vi "WPI_GyroAnalogOpen.vi"(6 "Calibrated Center Voltage":dbl, 7 "Calibration Time (s)":dbl=2.0, 8 "error in (no error)":errorcluster, 9 "Calibrate On Open":bool=TRUE, 10 "Analog Channel":T1) -> (0 "error out":errorcluster, 2 "Calibrated Center Voltage Out":dbl, 3 "GyroDevRef":T2={"DevStatus"={"status"=FALSE, "code"=0, "source"=""}, "Analog Channel"=enum."AI 1", "Gain (VoltsPerDegree/Second)"=0.0, "Gyro Type"=enum."Analog", "Handle"=0, "SPI Bus"=enum."Invalid", "Device Found"=FALSE, "Sample Rate"=1.0, "Calibrate On Open"=FALSE, "Offset"=0.0} {"Sample Rate" min=0.25 max=100.0 step=0.25})   [LabVIEW 2017]
doc: "Opens a reference to the gyroscope you specify. You must open a reference before using any other VIs on this palette.\n\nThis software is licensed. Open the labview\\readme\\WPI Robotics Library Open Source License.txt file for more information."
uses:
  <vilib>/Rock Robotics/WPI/Gyro/WPI_GyroDevRef.ctl
  <vilib>/Rock Robotics/SystemInterfaces/AI/FPGA_AIChannel.ctl
  <vilib>/Rock Robotics/SystemInterfaces/spilib/spi_bus.ctl
  <vilib>/Rock Robotics/SystemInterfaces/AI/FPGA_AIGyroChannel.ctl
  <vilib>/robotics/Simulator/Engine/ctl/DeviceID.ctl
  <instrlib>/Sparkfun Atomic IMU/HAIOL/Simulator/Sparkfun Atomic IMU Simulator.lvclass
  <vilib>/robotics/Simulator/NI_Robotics_Simulator.lvlib
  <instrlib>/Honeywell Compass HMC6343/HAIOL/Simulator/Honeywell Compass HMC6343 Simulator.lvclass
panel:
  # "Analog"
  # "XRS"
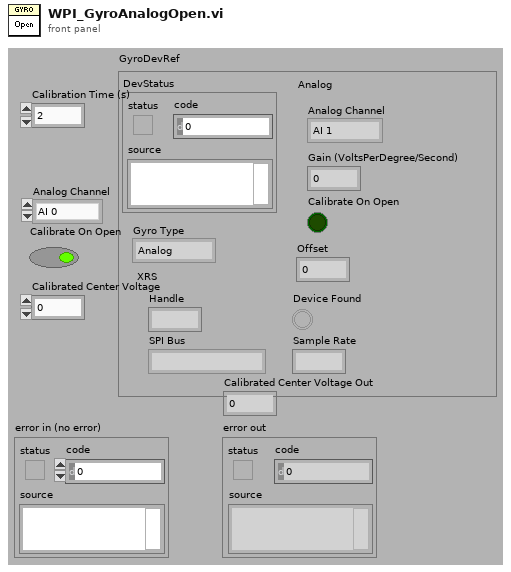
[diagram p1: front panel]
types:
  T1 = typedef "FPGA_AIGyroChannel.ctl" = enum8{"AI 0", "AI 1", "Invalid"}
  T2 = typedef "WPI_GyroDevRef.ctl" = cluster{"DevStatus":errorcluster, "Analog Channel":T3, "Gain (VoltsPerDegree/Second)":dbl, "Gyro Type":enum16{"Analog", "XRS450"}, "Handle":i32, "SPI Bus":T4, "Device Found":bool, "Sample Rate":dbl, "Calibrate On Open":bool, "Offset":dbl}
  T3 = typedef "FPGA_AIChannel.ctl" = enum8{"AI 0", "AI 1", "AI 2", "AI 3", "AI MXP 0", "AI MXP 1", "AI MXP 2", "AI MXP 3", "Invalid"}
  T4 = typedef "spi_bus.ctl" = enum16{"SPI On-Board, CS0", "SPI On-Board, CS1", "SPI On-Board, CS2", "SPI On-Board, CS3", "SPI MXP", "Invalid"}
  T5 = typedef "NI_Robotics_Simulator.lvlib/DeviceID.ctl" = cluster{"robot ID":string, "sensor/actuator ID":string}
  T6 = typedef "WPI_AnalogChannelDevRef.ctl" = cluster{"DevStatus":errorcluster, "Analog Channel":T3}
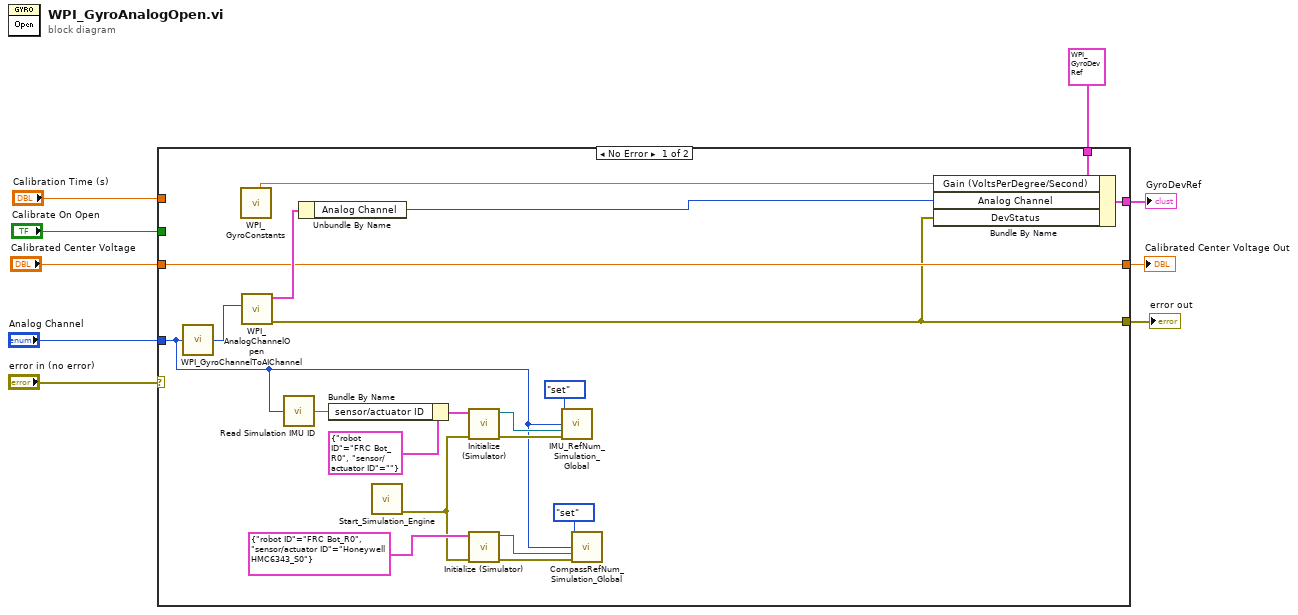
[diagram p0: block diagram]
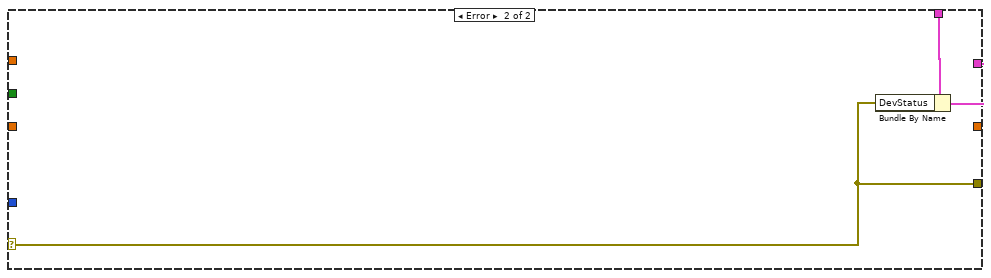
[diagram p2: hidden frame]
diagram:
  n1 = case shown="No Error" "error in (no error)" {
    selector: "error in (no error)" -> [_ w30]
    tunnel: "Analog Channel" -> [w15 _]
    tunnel: [w22 w30] -> w8
    tunnel: T2 {"DevStatus"={"status"=FALSE, "code"=0, "source"=""}, "Analog Channel"=enum."Invalid", "Gain (VoltsPerDegree/Second)"=0.0, "Gyro Type"=enum."Analog", "Handle"=0, "SPI Bus"=enum."Invalid", "Device Found"=FALSE, "Sample Rate"=1.0, "Calibrate On Open"=FALSE, "Offset"=0.0} ("GryoDevStatus") -> [w28 w31]
    tunnel: [w27 w32] -> w5
    tunnel: "Calibrate On Open" -> [_ _]
    tunnel: "Calibrated Center Voltage" -> [w23 _]
    tunnel: "Calibration Time (s)" -> [_ _]
    tunnel: [w23 _] -> w1
    frame No Error {
      n2 = call <vilib>:"WPI_GyroChannelToAIChannel.vi"("Gyro Channel"=w15) -> ("AI Channel"=w26:T3)  [unwired: 4 out]
      n3 = call <vilib>:"WPI_GyroConstants.vi"() -> ("Gain (VoltsPerDegreePerSecond)"=w24:dbl)  [unwired: 11 out]
      n4 = call <vilib>:"WPI_AnalogChannelOpen.vi"("Analog Channel"=w26) -> ("error out"=w22:errorcluster, "AIDeviceRef"=w25:T6)  [unwired: 2 in, 7 out]
      n5 = call <vilib>:"Read Simulation IMU ID.vi"("Analog Channel"=w15) -> ("gyro ID"=w19:string)  [unwired: 13 in, 1 out]
      n6 = Unbundle By Name(w25) -> ("Analog Channel"=w29:T3)
      n7 = Bundle By Name(cluster=T5 {"robot ID"="FRC Bot_R0", "sensor/actuator ID"=""} ("Device ID"), "sensor/actuator ID"=w19) -> (w20:T5)
      n8 = call <vilib>:"Start_Simulation_Engine.vi"() -> ("error out"=w13:errorcluster)  [unwired: 15 in]
      n9 = call <instrlib>:"Initialize (Simulator).vi"("error in (no error)"=w13, "Device ID"=w20) -> ("error out"=w16:errorcluster, "Sparkfun Atomic IMU out"=w18:refnum<class "Sparkfun Atomic IMU.lvclass">)  [unwired: 8 in]
      n10 = call <instrlib>:"Initialize (Simulator).vi"("error in (no error)"=w13, "Device ID"=T5 {"robot ID"="FRC Bot_R0", "sensor/actuator ID"="Honeywell HMC6343_S0"}) -> ("error out"=w11:errorcluster, "Honeywell Compass HMC6343"=w10:refnum<class "Honeywell Compass HMC6343.lvclass">)  [unwired: 8 in]
      n11 = call <vilib>:"IMU_RefNum_Simulation_Global.vi"("menu"=enum16{"set", "get", "delete"}."set", "Analog Channel"=w15, "Sparkfun Atomic IMU Set"=w18, "error in (no error)"=w16) -> ()  [unwired: 10 in, 2 out]
      n12 = call <vilib>:"CompassRefNum_Simulation_Global.vi"("menu"=enum16{"set", "get", "delete"}."set", "Analog Channel"=w15, "Honeywell Compass HMC6343 Set"=w10, "error in (no error)"=w11) -> ()  [unwired: 10 in, 2 out]
      n13 = Bundle By Name(cluster=w28, "Gain (VoltsPerDegree/Second)"=w24, "Analog Channel"=w29, "DevStatus"=w22) -> (w27:T2)
    }
    frame Error {
      n14 = Bundle By Name(cluster=w31, "DevStatus"=w30) -> (w32:T2)
    }
  }
  "GyroDevRef" <- w5
  "error out" <- w8
  "Calibrated Center Voltage Out" <- w1
